vi "Query Signaling TDD DL Flexible Slot Symbol.vi"(8 "error in (no error)":errorcluster, 9 "Pattern (1)":T1=1, 10 "Cell Name (\"Cell Name\")":string="Cell Name", 11 "VISA resource name":refnum<visa-resource-name>) -> (0 "error out":errorcluster, 2 "Slot Symbol":i32, 3 "VISA resource name out":refnum<visa-resource-name>)   [LabVIEW 2020, in "Rohde&Schwarz CMWXP NR FR1 Measurement.lvlib"]
doc: "Queries the number of DL symbols in the flexible slot of the UL-DL pattern <p>.\n\nAttribute:\n-\n\nRemote-control command:\n[CONFigure:]SIGNaling:NRADio:CELL:TDD:PATTern<p>:DL:FSSYmbol?"
uses:
  <instrlib>/Rohde&Schwarz CMWXP NR FR1 Measurement/Rohde&Schwarz CMWXP NR FR1 Measurement.lvlib
  <instrlib>/Rohde&Schwarz CMWXP NR FR1 Measurement/Private/_Pattern.ctl
  <instrlib>/Rohde&Schwarz CMWXP NR FR1 Measurement/Private/rsidr_core.llb/rsidr_core.lvlib
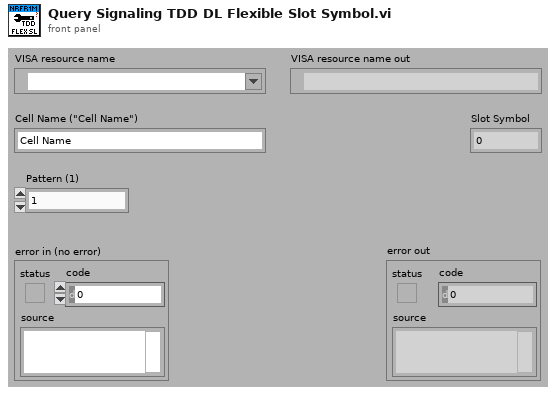
[diagram p1: front panel]
types:
  T1 = typedef "Rohde&Schwarz CMWXP NR FR1 Measurement.lvlib/_Pattern.ctl" = i32
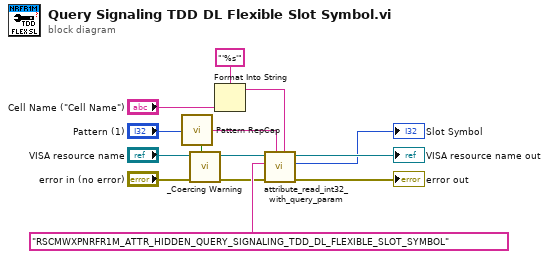
[diagram p0: block diagram]
diagram:
  n1 = call <instrlib>:"Pattern RepCap.vi"("Pattern In"="Pattern (1)") -> ("In Range?"=w4:bool, "RepCap Identifier Out"=w11:string)  [unwired: 1 in]
  n2 = call <instrlib>:"_Coercing Warning.vi"("In Range?"=w4, "error in (no error)"="error in (no error)", "VISA resource name"="VISA resource name") -> ("error out"=w6:errorcluster, "VISA resource name out"=w5:refnum<visa-resource-name>)  [unwired: 7 in]
  n3 = Format Into String(format string="'%s'", "Cell Name (\"Cell Name\")") -> (resulting string=w1:string)  [unwired: 2 in, 1 out]
  n4 = call <instrlib>:"attribute_read_int32_with_query_param.vi"("Query Parameter (None)"=w1, "Repeated Capability"=w11, "error in"=w6, "Attribute ID"="RSCMWXPNRFR1M_ATTR_HIDDEN_QUERY_SIGNALING_TDD_DL_FLEXIBLE_SLOT_SYMBOL", "VISA resource name"=w5) -> ("error out"=→"error out":errorcluster, "I32 out"=→"Slot Symbol":i32, "VISA resource name out"=→"VISA resource name out":refnum<visa-resource-name>)  [unwired: 4 in]
